vi "FTW-Connector-SpawnNewActor-Class.vi"(0 "FTW Actor Connector Type":refnum<class "FTW-ActorConnector.lvclass">, 5 "Configuration":string="{\n  \"Identity\": \"ActorName\",\n  \"DebugEnableInboxLogging\": false,\n  \"DebugEnableJobLogging\": false,\n  \"InboxAddress\": \"inproc://*\",\n  \"DebugShowPanel\": false\n}", 7 "Actor Instance":refnum<class "FTW-ActorInstance.lvclass">, 9 "Timeout":i32=-2 format="%dmsec", 11 "error in":errorcluster) -> (4 "FTW Actor Connector":refnum<class "FTW-ActorConnector.lvclass">, 6 "Initialized Response":string, 8 "Instance Inbox Address":string, 10 "Publishers":cluster{"Name":string, "URI":string}[](array[cluster]), 15 "error out":errorcluster)   [LabVIEW 2018, in "FTW-ActorConnector.lvclass"]
doc: "This is the spawn new actor that was used for a while. It lacks the minimum strict inputs required to launch an actor."
uses:
  FTW-ActorConnector.lvclass
  Instance/FTW-ActorInstance.lvclass
panel:
  # "Inputs"
  # "Outputs"
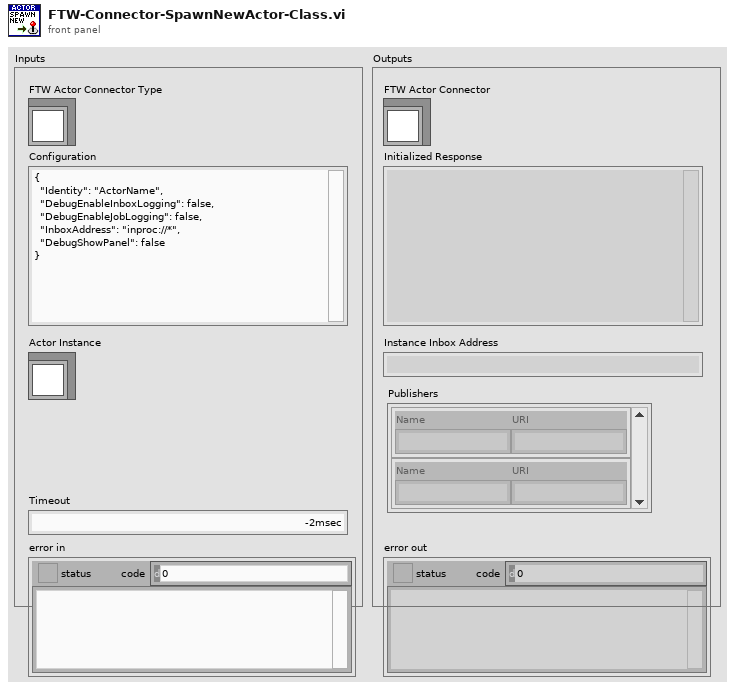
[diagram p1: front panel]
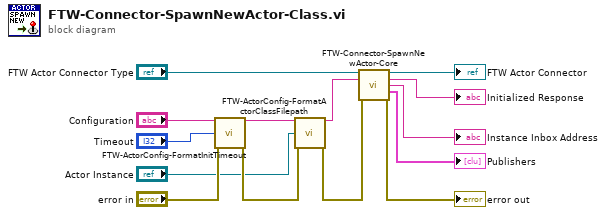
[diagram p0: block diagram]
diagram:
  n1 = call "FTW-ActorConfig-FormatInitTimeout.vi"("FTW Config String In"="Configuration", "Init Timeout"="Timeout", "error in"="error in") -> ("FTW Config String"=w7:string, "error out"=w5:errorcluster)  [unwired: 11 in]
  n2 = call "FTW-ActorConfig-FormatActorClassFilepath.vi"("FTW Config String In"=w7, "Actor Instance"="Actor Instance", "error in"=w5) -> ("FTW Config String"=w6:string, "error out"=w4:errorcluster)  [unwired: 11 in]
  n3 = call "FTW-Connector-SpawnNewActor-Core.vi"("FTW Actor Connector Type"="FTW Actor Connector Type", "Configuration"=w6, "error in"=w4) -> ("FTW Actor Connector"=→"FTW Actor Connector":refnum<class "FTW-ActorConnector.lvclass">, "Initialized Response"=→"Initialized Response":string, "Instance Inbox Address"=→"Instance Inbox Address":string, "Publishers"=→"Publishers":cluster{"Name":string, "URI":string}[], "error out"=→"error out":errorcluster)  [unwired: 8 in]
